vi "grabber essentials panel.vi"() -> ()   [LabVIEW 2010]
panel:
  in  "close stage":bool
  in  "open stage":bool
  in  "engage stage feedback":bool
  in  "gaussian":bool
  in  "r sphere/sigma (um)":dbl=3.0
  in  "reset tracker":bool
  in  "tracking?":bool
  in  "Pockels cell bleach":i16=100 min=-750 max=750 step=1
  in  "spilt ff/fb":bool
  in  "Pockels cell voltage":i16=60 min=-750 max=750 step=1
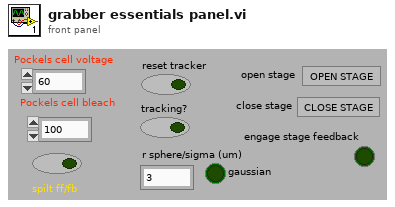
[diagram p1: front panel]
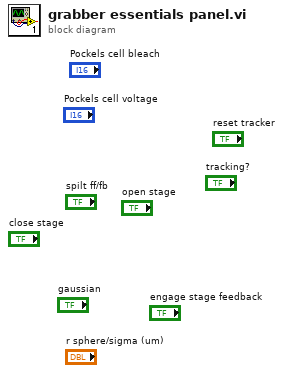
[diagram p0: block diagram]
diagram:
